vi "emi_Control enable and visibility array.vi"(0 "Controls":refnum<vi>[](array[refnum]), 7 "State(Normal)":enum16{"Normal", "Disabled", "Grayed", "Hidden"}(ring), 11 "error in":errorcluster) -> (4 "Constrols out":refnum<vi>[](array[refnum]), 15 "error out":errorcluster)   [LabVIEW 2011]
doc: "Set state: Normal, Disabled, Grayed, hidden of array of controls.\n\nOn error: Does nothing."
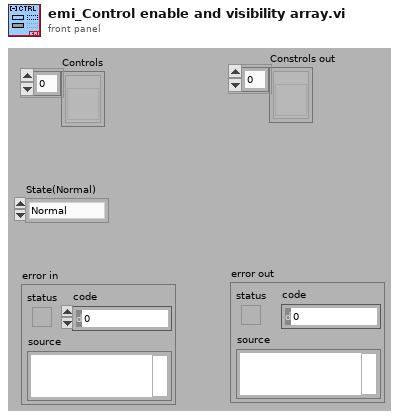
[diagram p1: front panel]
types:
  T1 = enum8{"Enabled", "Disabled", "Disabled and Grayed Out"}
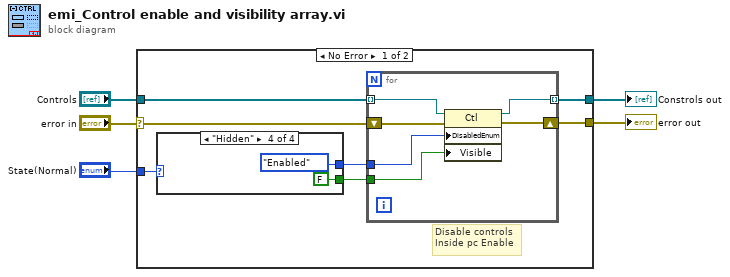
[diagram p0: block diagram]
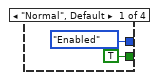
[diagram p2: hidden frame]
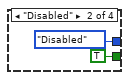
[diagram p3: hidden frame]
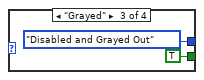
[diagram p4: hidden frame]
diagram:
  n1 = case shown="No Error" "error in" {
    selector: "error in" -> [w6 w28]
    tunnel: [w12 w27] -> w5
    tunnel: "Controls" -> [w11 w27]
    tunnel: [w10 w28] -> w3
    tunnel: "State(Normal)" -> [w9 _]
    frame No Error {
      # "Disable controls\nInside pc Enable"
      n2 = case shown="\"Hidden\"" w9 {
        tunnel: [T1."Enabled" ("Disabled") T1."Disabled" ("Disabled") T1."Disabled and Grayed Out" ("Disabled") T1."Enabled" ("Disabled")] -> w8
        tunnel: [TRUE TRUE TRUE FALSE] -> w7
        frame "Normal", Default {
        }
        frame "Disabled" {
        }
        frame "Grayed" {
        }
        frame "Hidden" {
        }
      }
      n3 = for {
        tunnel: w11 -> [w25] mode=indexing
        tunnel: w8 -> [w24]
        tunnel: [w22] -> w12 mode=indexing
        tunnel: w7 -> [w21]
        shift-right: [w23] -> w10
        shift-left: w6 -> [w26]
        n4 = property class="Ctl"(reference=w25, error in=w26, "DisabledEnum"=w24, "Visible"=w21) -> (reference out=w22:refnum<vi>, error out=w23:errorcluster)
      }
    }
    frame Error {
    }
  }
  "Constrols out" <- w5
  "error out" <- w3
